vi "Calculate normal moves.vi"(7 "Position in":refnum<class "Position.lvclass">, 11 "Source":T1) -> (3 "Normal moves":refnum<class "CastleRestricting.lvclass">[](array[class]))   [LabVIEW 2016, in "Chesslib.lvlib" / "King.lvclass"]
uses:
  King.lvclass
  Moves/CastleRestricting/CastleRestricting.lvclass
  Position/Position.lvclass
  typedef/Square.ctl
  typedef/File.ctl
  typedef/Rank.ctl
  typedef/Neighbor.ctl
  Chesslib.lvlib
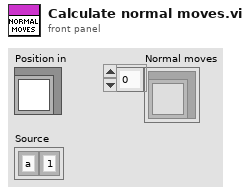
[diagram p1: front panel]
types:
  T1 = typedef "Chesslib.lvlib/Square.ctl" = cluster{"File":T2, "Rank":T3}
  T2 = typedef "Chesslib.lvlib/File.ctl" = enum8{"a", "b", "c", "d", "e", "f", "g", "h"}
  T3 = typedef "Chesslib.lvlib/Rank.ctl" = enum8{"1", "2", "3", "4", "5", "6", "7", "8"}
  T4 = typedef "Chesslib.lvlib/Neighbor.ctl" = enum16{"N", "NW", "W", "SW", "S", "SE", "E", "NE", "vector"}
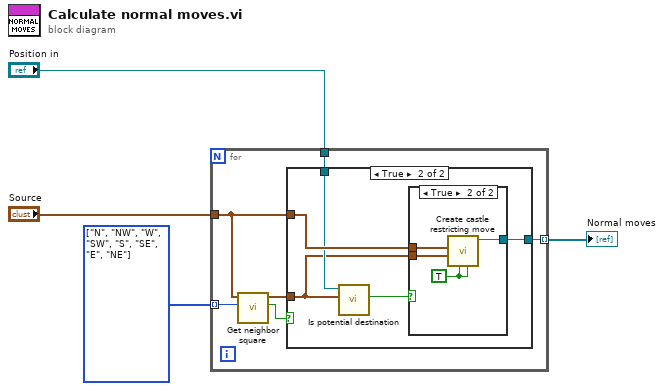
[diagram p0: block diagram]
diagram:
  w2 = T4[] [enum."N", enum."NW", enum."W", enum."SW", enum."S", enum."SE", enum."E", enum."NE"] items=["N", "NW", "W", "SW", "S", "SE", "E", "NE", "vector"]
  n1 = for {
    tunnel: "Source" -> [w7]
    tunnel: w2 -> [w10] mode=indexing
    tunnel: "Position in" -> [w6]
    tunnel: [w5] -> w4 mode=indexing
    n2 = call "Get neighbor square.vi"("Neighbor (vector)"=w10, "Square in"=w7) -> ("Valid"=w9:bool, "Square out"=w8:T1)  [unwired: 7 in, 1 out]
    n3 = case shown="True" w9 {
      tunnel: w8 -> [_ w12]
      tunnel: w7 -> [_ w15]
      tunnel: w6 -> [_ w13]
      tunnel: [_ w14] -> w5
      frame False {
      }
      frame True {
        n4 = call "Is potential destination.vi"("Square"=w12, "Position in"=w13) -> ("Potential destination"=w11:bool)  [unwired: 7 in, 2 out]
        n5 = case shown="True" w11 {
          tunnel: w15 -> [_ w19]
          tunnel: w12 -> [_ w18]
          tunnel: [_ w17] -> w14
          frame False {
          }
          frame True {
            w16 = TRUE ("Restrict king side")
            n6 = call "Create castle restricting move.vi"("Restrict queen side (F)"=w16, "Restrict king side (F)"=w16, "Destination"=w18, "Source"=w19) -> ("CastleRestricting out"=w17:refnum<class "CastleRestricting.lvclass">)  [unwired: 6 in, 1 out]
          }
        }
      }
    }
  }
  "Normal moves" <- w4
